vi "Encoder Position & Velocity (FPGA).vi"(3 "Velocity Interval (uSec)":u32=1000, 5 "Position Reset":bool) -> (0 "Velocity (Counts/Interval)":i32, 1 "Acceleration (Counts/Interval)":i32, 2 "Position (Counts)":i32)   [LabVIEW 2009]
doc: "This is an FPGA vi for Quadrature Encoder Velocity and Acceleration Estimation using CompactRIO. It requires as inputs a Fixed Time Interval for velocity and acceleration estimation.\n\nThis application is designed to work with an R-Series expansion setup using PCI/PXI-7811R FPGA device and a CompactRIO cRIO-9411 digital input module installed in slot 1 of the expansion chassis."
uses:
  <vilib>/rvi/Arithmetic/AddSubMult/XNode/nirviSatArithmetic.xnode
  <vilib>/eio/EIONode/EIONode.xnode
  <vilib>/rvi/eio/nirviEIOImplementation/nirviEIOImplementation.xnode
  <vilib>/rvi/eio/common/nirviEmuTemplateMethod_noerrors.vi
  <vilib>/rvi/eio/common/nirviEmuClasses.ctl
panel:
  in  "stop":bool
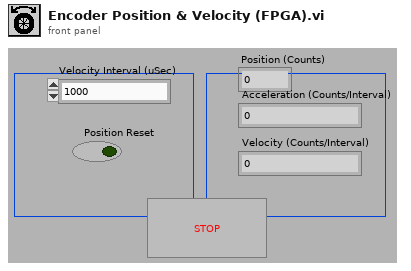
[diagram p1: front panel]
types:
  T1 = typedef "nirviEmuClasses.ctl" = enum16{"IO Read", "IO Write", "Method", "Property Read", "Property Write"}
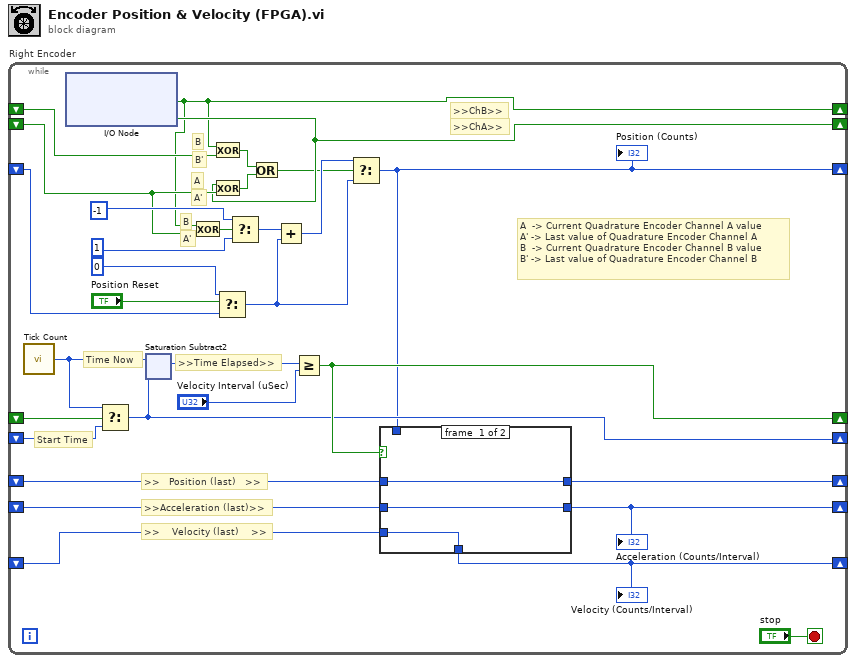
[diagram p0: block diagram]
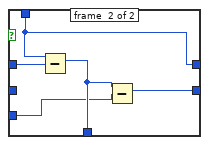
[diagram p2: hidden frame]
diagram:
  n1 = while "Right Encoder" {
    shift-right: [w1] -> _
    shift-left: _ -> [w6]
    shift-right: [w5] -> _
    shift-left: _ -> [w17]
    shift-right: [w20] -> _
    shift-left: _ -> [w21]
    shift-right: [w13] -> _
    shift-left: _ -> [w16]
    shift-right: [w8] -> _
    shift-left: _ -> [w14]
    shift-right: [w2] -> _
    shift-left: _ -> [w11]
    shift-right: [w3] -> _
    shift-left: _ -> [w10]
    shift-right: [w4] -> _
    shift-left: _ -> [w7]
    stop <- "stop" stop-if-true
    # "A  -> Current Quadrature Encoder Channel A value\nA' -> Last value of Quadrature Encoder Channel A\nB  -> Current Quadrature Encoder Channel B value\nB' -> Last value of Quadrature Encoder Channel B"
    # ">>Acceleration (last)>>"
    # "Start Time"
    # "A'"
    # "B"
    # "A'"
    # "A"
    # "B'"
    # "B"
    # ">>ChB>>"
    # ">>ChA>>"
    # ">>    Velocity (last)    >>"
    # ">>   Position (last)   >>"
    # "Time Now"
    # ">>Time Elapsed>>"
    n2 = call "Tick Count"() -> ("Tick Count(uSec)"=w9:u32)
    n3 = xnode "I/O Node"() -> ("Mod2/DIO10"=w1:bool, "Mod2/DIO9"=w20:bool)  [unwired: 2 in, 2 out]
    n4 = Select(t=w9, s=w16, f=w14) -> (s? t:f=w8:u32)
    n5 = xnode ("Saturation Subtract2")("x"=w9, "y"=w8) -> ("x-y"=w12:u32)
    n6 = Exclusive Or(1:w21, 2:w1) -> (0:w22:bool)
    n7 = Exclusive Or(1:w6, 2:w1) -> (0:w23:bool)
    n8 = Exclusive Or(1:w21, 2:w20) -> (0:w24:bool)
    n9 = Select(t=0 ("32 bit"), s="Position Reset", f=w17) -> (s? t:f=w29:i32)
    n10 = Select(t=-1 ("32 bit"), s=w22, f=1 ("32 bit")) -> (s? t:f=w27:i32)
    n11 = Or(x=w23, y=w24) -> (x .or. y?=w18:bool)
    n12 = Add(x=w27, y=w29) -> (x+y=w31:i32)
    n13 = Greater Or Equal?(x=w12, y="Velocity Interval (uSec)") -> (x >= y?=w13:bool)
    n14 = Select(t=w31, s=w18, f=w29) -> (s? t:f=w5:i32)
    "Position (Counts)" <- w5
    n15 = case shown="True" w13 {
      tunnel: w5 -> [_ w83]
      tunnel: w11 -> [w80 w87]
      tunnel: [w82 w86] -> w3
      tunnel: w10 -> [w82 w85]
      tunnel: [w81 w84] -> w4
      tunnel: w7 -> [w81 _]
      tunnel: [w80 w83] -> w2
      frame #0 {
      }
      frame #1 {
        n16 = Subtract(x=w83, y=w87) -> (x-y=w86:i32)
        n17 = Subtract(x=w86, y=w85) -> (x-y=w84:i32)
      }
    }
    "Acceleration (Counts/Interval)" <- w4
    "Velocity (Counts/Interval)" <- w3
  }
